vi "DataLog Basic Logging.vi"() -> (0 "pass?":bool)   [LabVIEW 2012]
panel:
  in  "script file":path=path "scripts/basic logging.lua"
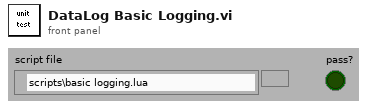
[diagram p1: front panel]
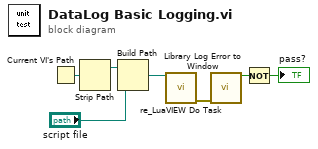
[diagram p0: block diagram]
diagram:
  n1 = Current VI's Path() -> (path=w4:path)
  n2 = Strip Path(path=w4) -> (stripped path=w3:path)  [unwired: 1 out]
  n3 = Build Path(base path=w3, name or relative path="script file") -> (appended path=w1:path)
  n4 = call "re_LuaVIEW Do Task.vi"("script file or name (no name)"=w1) -> ("error out"=w5:errorcluster)  [unwired: 14 in]
  n5 = call "Library Log Error to Window.vi"("error in (no error)"=w5) -> ("error?"=w7:bool)  [unwired: 13 in, 1 out]
  n6 = Not(x=w7) -> (.not. x?=→"pass?":bool)
